vi "Set plotnames2.vi"(8 "error in (no error)":errorcluster caption="에러 입력(에러 없음)", 10 "플롯 이름":string[](array[string]), 11 "그래프 참조":refnum<vi>) -> (0 "error out":errorcluster caption="에러 출력")   [LabVIEW 2018]
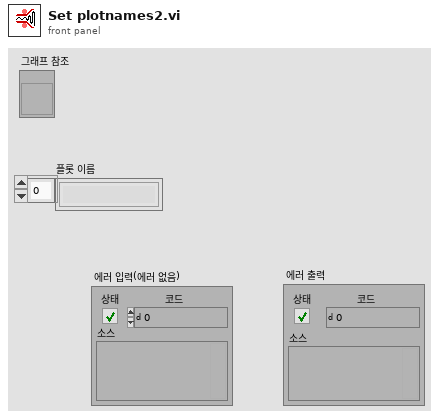
[diagram p1: front panel]
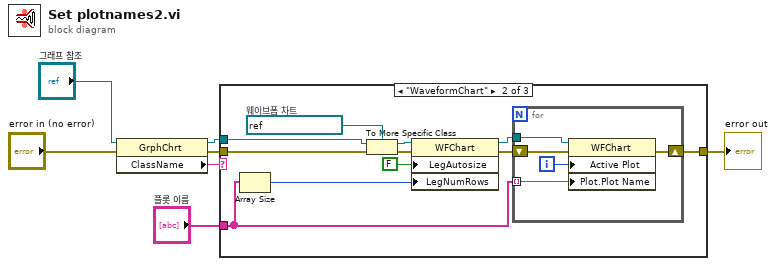
[diagram p0: block diagram]
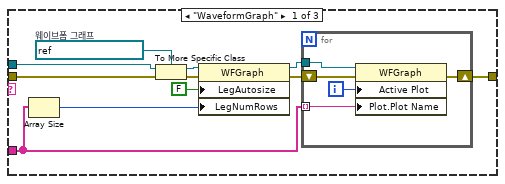
[diagram p2: hidden frame]
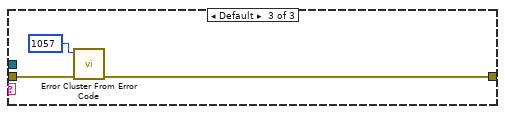
[diagram p3: hidden frame]
diagram:
  n1 = property class="GrphChrt"(reference="그래프 참조", error in="error in (no error)") -> (reference out=w5:refnum<vi>, error out=w4:errorcluster, "ClassName"=w2:string)
  n2 = case "케이스 구조" shown="\"WaveformChart\"" w2 {
    tunnel: w5 -> [w18 w34 _]
    tunnel: w4 -> [w17 w33 w42]
    tunnel: "플롯 이름" -> [w12 w28 _]
    tunnel: [w8 w24 w40] -> w1
    frame "WaveformGraph" {
      w16 = refnum<vi> refnum  # 웨이브폼 그래프
      n3 = Array Size(array=w12) -> (size(s)=w11:i32)
      n4 = To More Specific Class(target class=w16, reference=w18, error in=w17) -> (specific class reference=w15:refnum<vi>, error out=w10:errorcluster)
      n5 = property class="WFGraph"(reference=w15, error in=w10, "LegAutosize"=FALSE ("범례:자동 크기 조정"), "LegNumRows"=w11) -> (reference out=w13:refnum<vi>, error out=w9:errorcluster)
      n6 = for {
        tunnel: w13 -> [w23]
        tunnel: w12 -> [w22] mode=indexing
        shift-right: [w19] -> w8
        shift-left: w9 -> [w20]
        i -> [w21]
        n7 = property class="WFGraph"(reference=w23, error in=w20, "Active Plot"=w21, "Plot.Plot Name"=w22) -> (error out=w19:errorcluster)  [unwired: 1 out]
      }
    }
    frame "WaveformChart" {
      w32 = refnum<vi> refnum  # 웨이브폼 차트
      n8 = Array Size(array=w28) -> (size(s)=w27:i32)
      n9 = To More Specific Class(target class=w32, reference=w34, error in=w33) -> (specific class reference=w31:refnum<vi>, error out=w26:errorcluster)
      n10 = property class="WFChart"(reference=w31, error in=w26, "LegAutosize"=FALSE ("범례:자동 크기 조정"), "LegNumRows"=w27) -> (reference out=w29:refnum<vi>, error out=w25:errorcluster)
      n11 = for {
        tunnel: w29 -> [w39]
        tunnel: w28 -> [w38] mode=indexing
        shift-right: [w35] -> w24
        shift-left: w25 -> [w36]
        i -> [w37]
        n12 = property class="WFChart"(reference=w39, error in=w36, "Active Plot"=w37, "Plot.Plot Name"=w38) -> (error out=w35:errorcluster)  [unwired: 1 out]
      }
    }
    frame Default {
      n13 = call <vilib>:"Error Cluster From Error Code.vi"("error in (no error)"=w42, "error code (0)"=1057) -> ("error out"=w40:errorcluster)  [unwired: 7 in]
    }
  }
  "error out" <- w1
